vi "list_tables.vi"(8 "error in (no error)":errorcluster, 11 "Doc in":refnum<class "Doc.lvclass">) -> (0 "error out":errorcluster, 2 "table_names":string[](array[string]), 3 "Doc out":refnum<class "Doc.lvclass">)   [LabVIEW 2020, in "toml_edit.lvlib" / "Doc.lvclass"]
uses:
  Doc.lvclass
  Doc.lvclass/Doc.ctl
  dragon_toml_64.dll
  toml_edit.lvlib
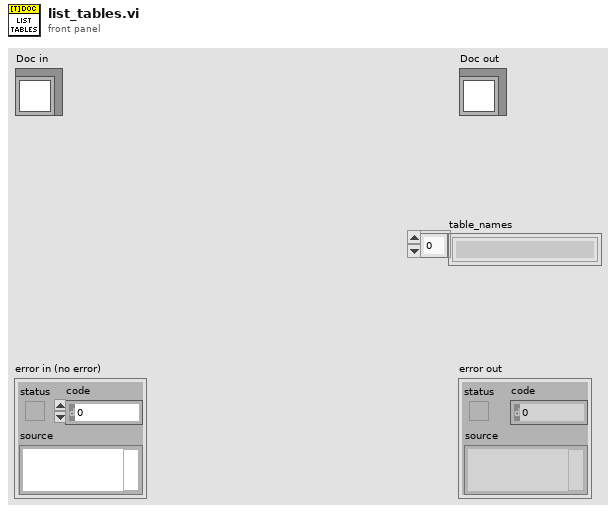
[diagram p1: front panel]
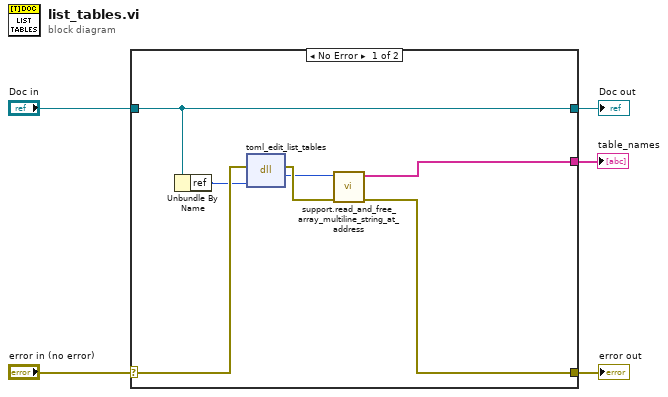
[diagram p0: block diagram]
diagram:
  n1 = case shown="No Error" "error in (no error)" {
    selector: "error in (no error)" -> [w10 w14]
    tunnel: [w8 w14] -> w4
    tunnel: [w7 w13] -> w2
    tunnel: "Doc in" -> [w7 w13]
    tunnel: [w9 _] -> w1
    frame No Error {
      n2 = Unbundle By Name(w7) -> ("ref"=w6:u64)
      n3 = dll-call lib="C:/Projects/toml-edit-labview/lv_src/dragon_toml_*.dll" fn="toml_edit_list_tables"(error in=w10, "doc_ref"=w6) -> (error out=w12:errorcluster, "table_names_ptr"=w11:u64)  [unwired: 3 in, 1 out]
      n4 = call "support.read_and_free_array_multiline_string_at_address.vi"("error in (no error)"=w12, "table_names_ptr"=w11) -> ("error out"=w8:errorcluster, "lines"=w9:string[])  [unwired: 8 in]
    }
    frame Error {
    }
  }
  "error out" <- w4
  "Doc out" <- w2
  "table_names" <- w1
